vi "Main.vi"(11 "Module Admin":refnum<class "Delacor_lib_QMH_Module Admin.lvclass">) -> ()   [LabVIEW 2021, in "Test Configuration.lvlib"]
doc: "This template is based off of the Queued Message Handler design pattern and the Queued Message Handler project template that ships with LabVIEW.\n\nThe main difference is that the queue is private to this module and communication between modules is performed via Broadcast and Request events.\n\nRequest events are wrapped in public API methods and are handled in the Event Handling Loop (EHL) of this VI. Any module can register for Broadcast events sent by this module. The EHL generates messages based on user interface actions.\n\nThe Message Handling Loop (MHL) processes messages generated by the EHL, or by other messages. The messages are string values, so new messages can be added easily to the Message Cases case structure in the MHL. Each message cluster can also provide an optional value for Message Data, which is a variant that can be converted to whatever message-specific data is required.\n_____\nBased on DQMH Project Template 7.0.1.1316."
uses:
  Test Configuration.lvlib
  <vilib>/Delacor/Delacor QMH/Libraries/Module Admin_class/Delacor_lib_QMH_Module Admin.lvclass
  Module Data--cluster.ctl
  <vilib>/Wovalab/Utilities/Helper Loop Periodic Timing/Helper Loop Periodic Timing.lvclass/Helper Loop Periodic Timing.ctl
  Host-Control's/Module ID Action Enum.ctl
  <vilib>/Delacor/Delacor QMH/Libraries/Message Queue_class/Delacor_lib_QMH_Message Queue.lvclass/Delacor_lib_QMH_Message Queue.ctl
  Stop Argument--cluster.ctl
  <vilib>/Delacor/Delacor QMH/Libraries/Module Admin_class/Delacor_lib_QMH_Module Admin.lvclass/Delacor_lib_QMH_Module Admin.ctl
  <vilib>/Utility/miscctls.llb/LVPointTypeDef.ctl
  Host-Control's/DTT Test folder Name's.ctl
  <vilib>/Delacor/Delacor QMH/Libraries/Message Queue_class/Delacor_lib_QMH_Enqueue Message (Single).vi
  <vilib>/Delacor/Delacor QMH/Libraries/Module Admin_class/Delacor_lib_QMH_Get External Launch.vi
  <vilib>/Wovalab/Utilities/Helper Loop Periodic Timing/U32 Max Value--constant.vi
  <vilib>/Wovalab/Utilities/Helper Loop Periodic Timing/Update Last Execution Time.vi
  <vilib>/Utility/traverseref.llb/TRef Get All FP References.vi
  <vilib>/Utility/traverseref.llb/Get GObject Label.vi
  <vilib>/Wovalab/Utilities/Helper Loop Periodic Timing/Helper Loop Periodic Timing.lvclass
  <vilib>/Delacor/Delacor QMH/Libraries/Message Queue_class/Delacor_lib_QMH_Message Queue.lvclass
  Main-Module/Host Main.lvlib
  RT Acquisition Engine/RT Acquisition Engine.lvlib
  <userlib>/_OpenG.lib/appcontrol/appcontrol.llb/openg_application_control.lvlib
panel:
  in  "Proceed":bool
  in  "Open Auto-Seq Config File":bool
  out "Auto Sequence Configuration File":path
  in  "Open sb-RIO Config Folder":bool
  out "Airbag Configuration File":path
  in  "Open Crio Config Folder":bool
  out "Capsule Configuration File":path
  out "Capsule-3":bool
  out "Capsule-4":bool
  out "Capsule-2":bool
  in  "Auto ?":bool
  in  "EM valve Delay (mS)":u32=1000
  out "sb-RIO":bool
  out "Capsule-1":bool
  out "Release":bool
  out "Safety":bool
  in  "Hardware Status check":bool
  in  "Gate valve Delay (mS)":u32=1000
  in  "Data Logging Duration (Sec)":dbl=20.0 min=10.0 max=70.0
  out "error out":errorcluster
  out "Status":string
  in  "Simulate MHL Error":bool
  in  "Simulate EHL Error":bool
  # "IIT M Drop Tower Test System"
  # "TEST CONFIGURATION"
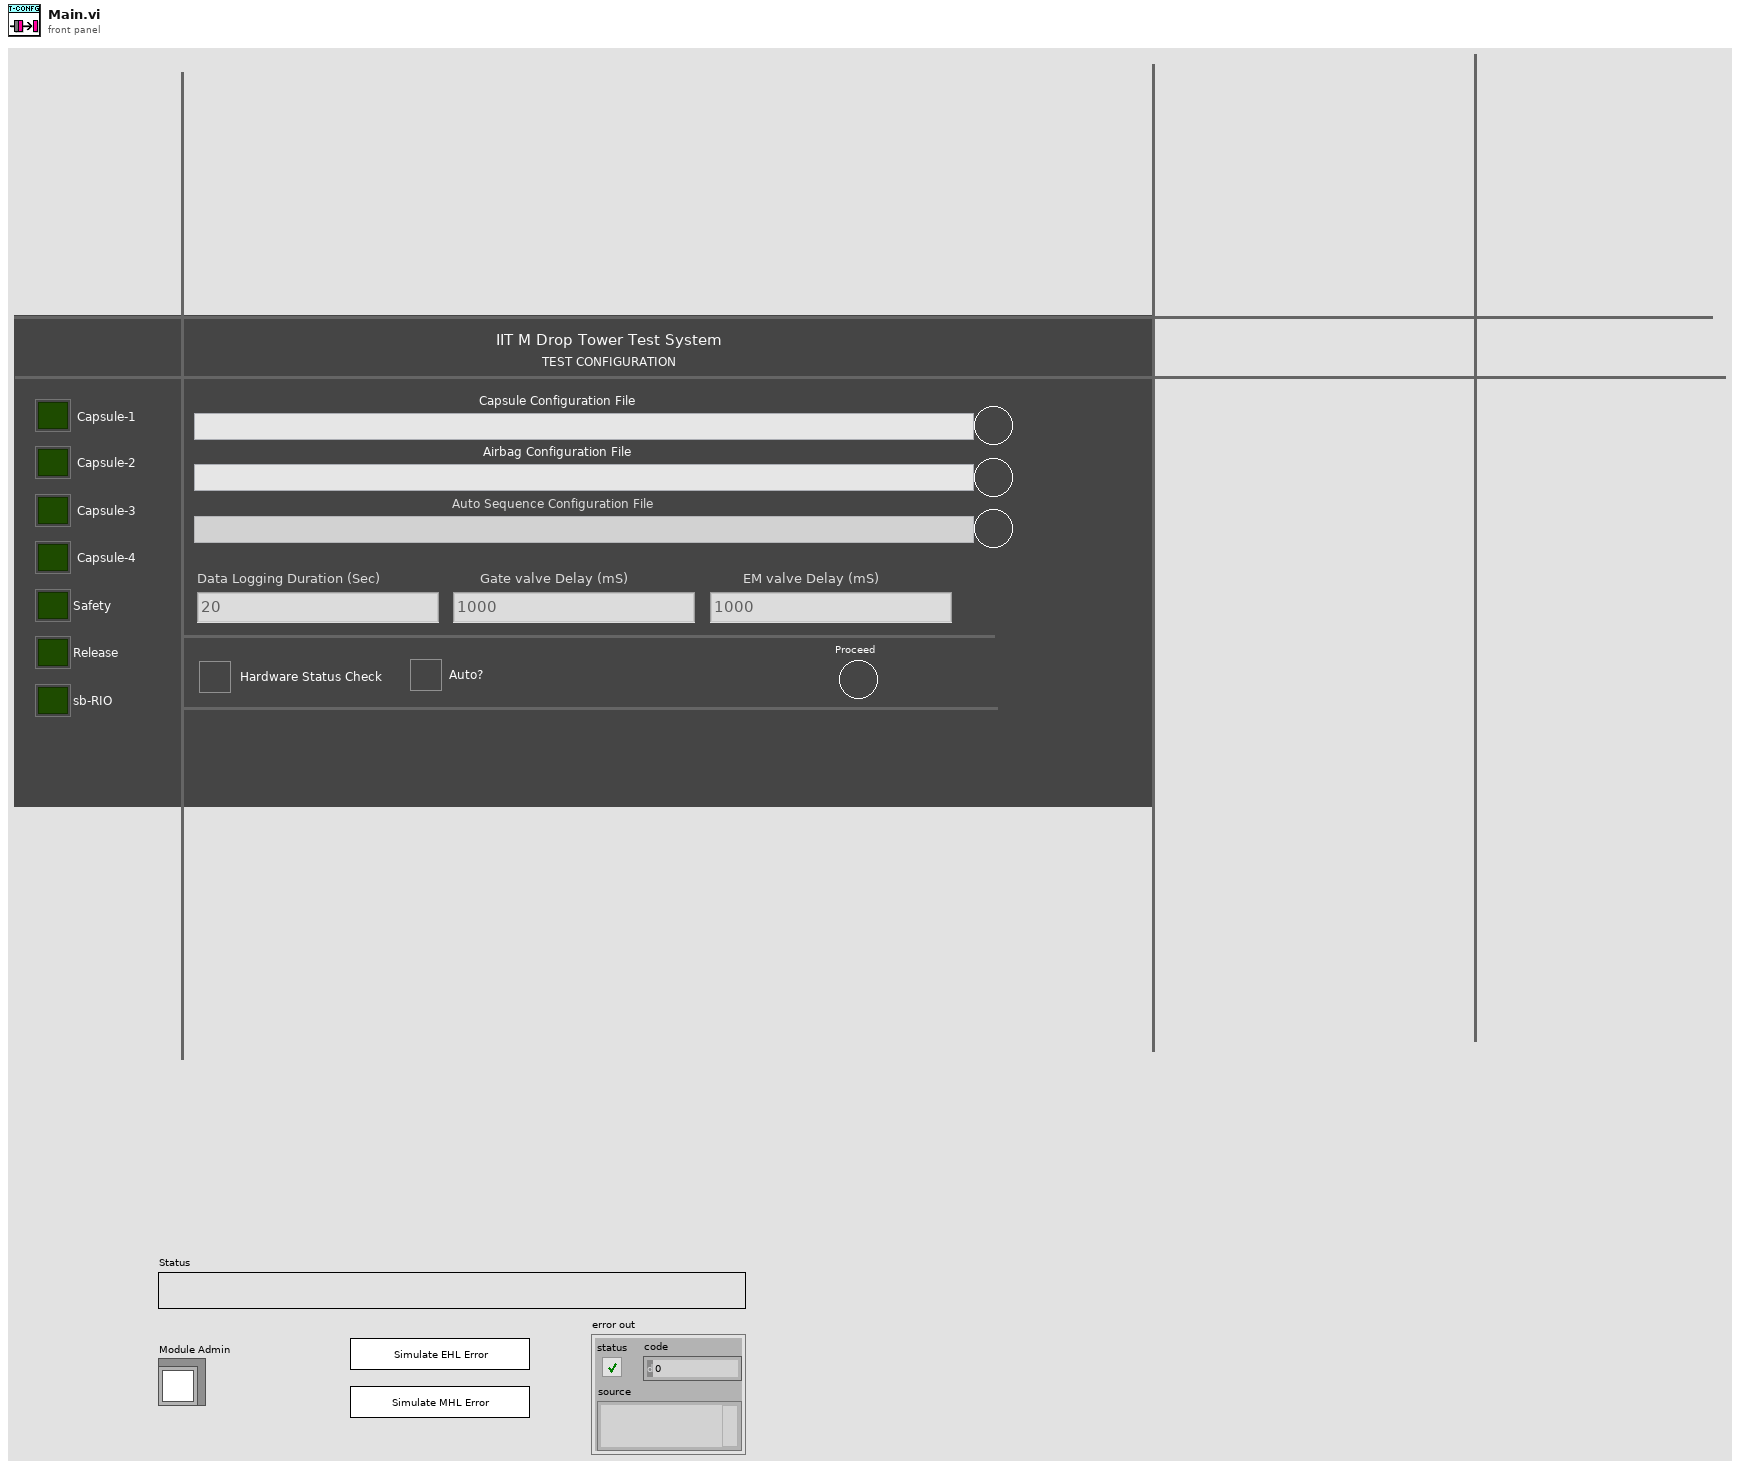
[diagram p1: front panel]
types:
  T1 = typedef "Test Configuration.lvlib/Request Events--cluster.ctl" = cluster{"Stop Module":refnum<user-event>, "Show Panel":refnum<user-event>, "Hide Panel":refnum<user-event>, "Get Module Execution Status":refnum<user-event>, "Show Diagram":refnum<user-event>}
  T2 = typedef "Test Configuration.lvlib/Module Data--cluster.ctl" = cluster{"Status":string, "Channel config Stating Path":path, "Auto-Seq config Stating Path":path, "c-RIO Tx Data":cluster{"cRIO-Module ID":i32, "AI-Config Data":string[], "AO-Config Data":string[], "DI-Config Data":string[], "DO-Config Data":string[], "AI-Start Cmd":string[], "AO-Start Cmd":string[], "DI-Start Cmd":string[], "DO-Start Cmd":string[], "AS Config Cmd":string}, "Auto Sequence Selected?":bool, "This VI":refnum<vi>, "GUI Data's":cluster{"All Object Ref":refnum<vi>[], "All Object Label":string[]}}
  T3 = typedef "Module ID Action Enum.ctl" = enum16{"Init", "Insert", "Get a ID", "Get all ID"}
  T4 = enum32{"invalid lock state", "Not Locked", "Locked (No Password)", "Password-protected"}
  T5 = typedef "Test Configuration.lvlib/Stop Argument--cluster.ctl" = cluster{"Origin":string, "Exit via Stop Module Req?":bool, "Wait for Module to stop?":bool}
  T6 = typedef "LVPointTypeDef.ctl" = cluster{"Horizontal":i16, "Vertical":i16}
  T7 = enum32{"Invalid", "Standard", "Closed", "Hidden", "Minimized", "Maximized"}
  T8 = typedef "DTT Test folder Name's.ctl" = enum16{"Event Log", "Auto Sequence Configuration", "Channel Configuration's", "Test Data's"}
  T9 = enum8{"Enabled", "Disabled", "Disabled and Grayed Out"}
  T10 = typedef "RT Acquisition Engine.lvlib/Broadcast Events--cluster.ctl" = cluster{"Module Did Init":refnum<user-event>, "Status Updated":refnum<user-event>, "Error Reported":refnum<user-event>, "Module Did Stop":refnum<user-event>, "Update Module Execution Status":refnum<user-event>, "RT Connection Status":refnum<user-event>, "Tx RT Hardware Info":refnum<user-event>, "DO Data's":refnum<user-event>, "AI-Info":refnum<user-event>, "Logging Completed":refnum<user-event>}
  T11 = typedef "HW Name Enum.ctl" = enum16{"Capsule-1", "Capsule-2", "Capsule-3", "Capsule-4", "sb-RIO", "Safety", "Release"}
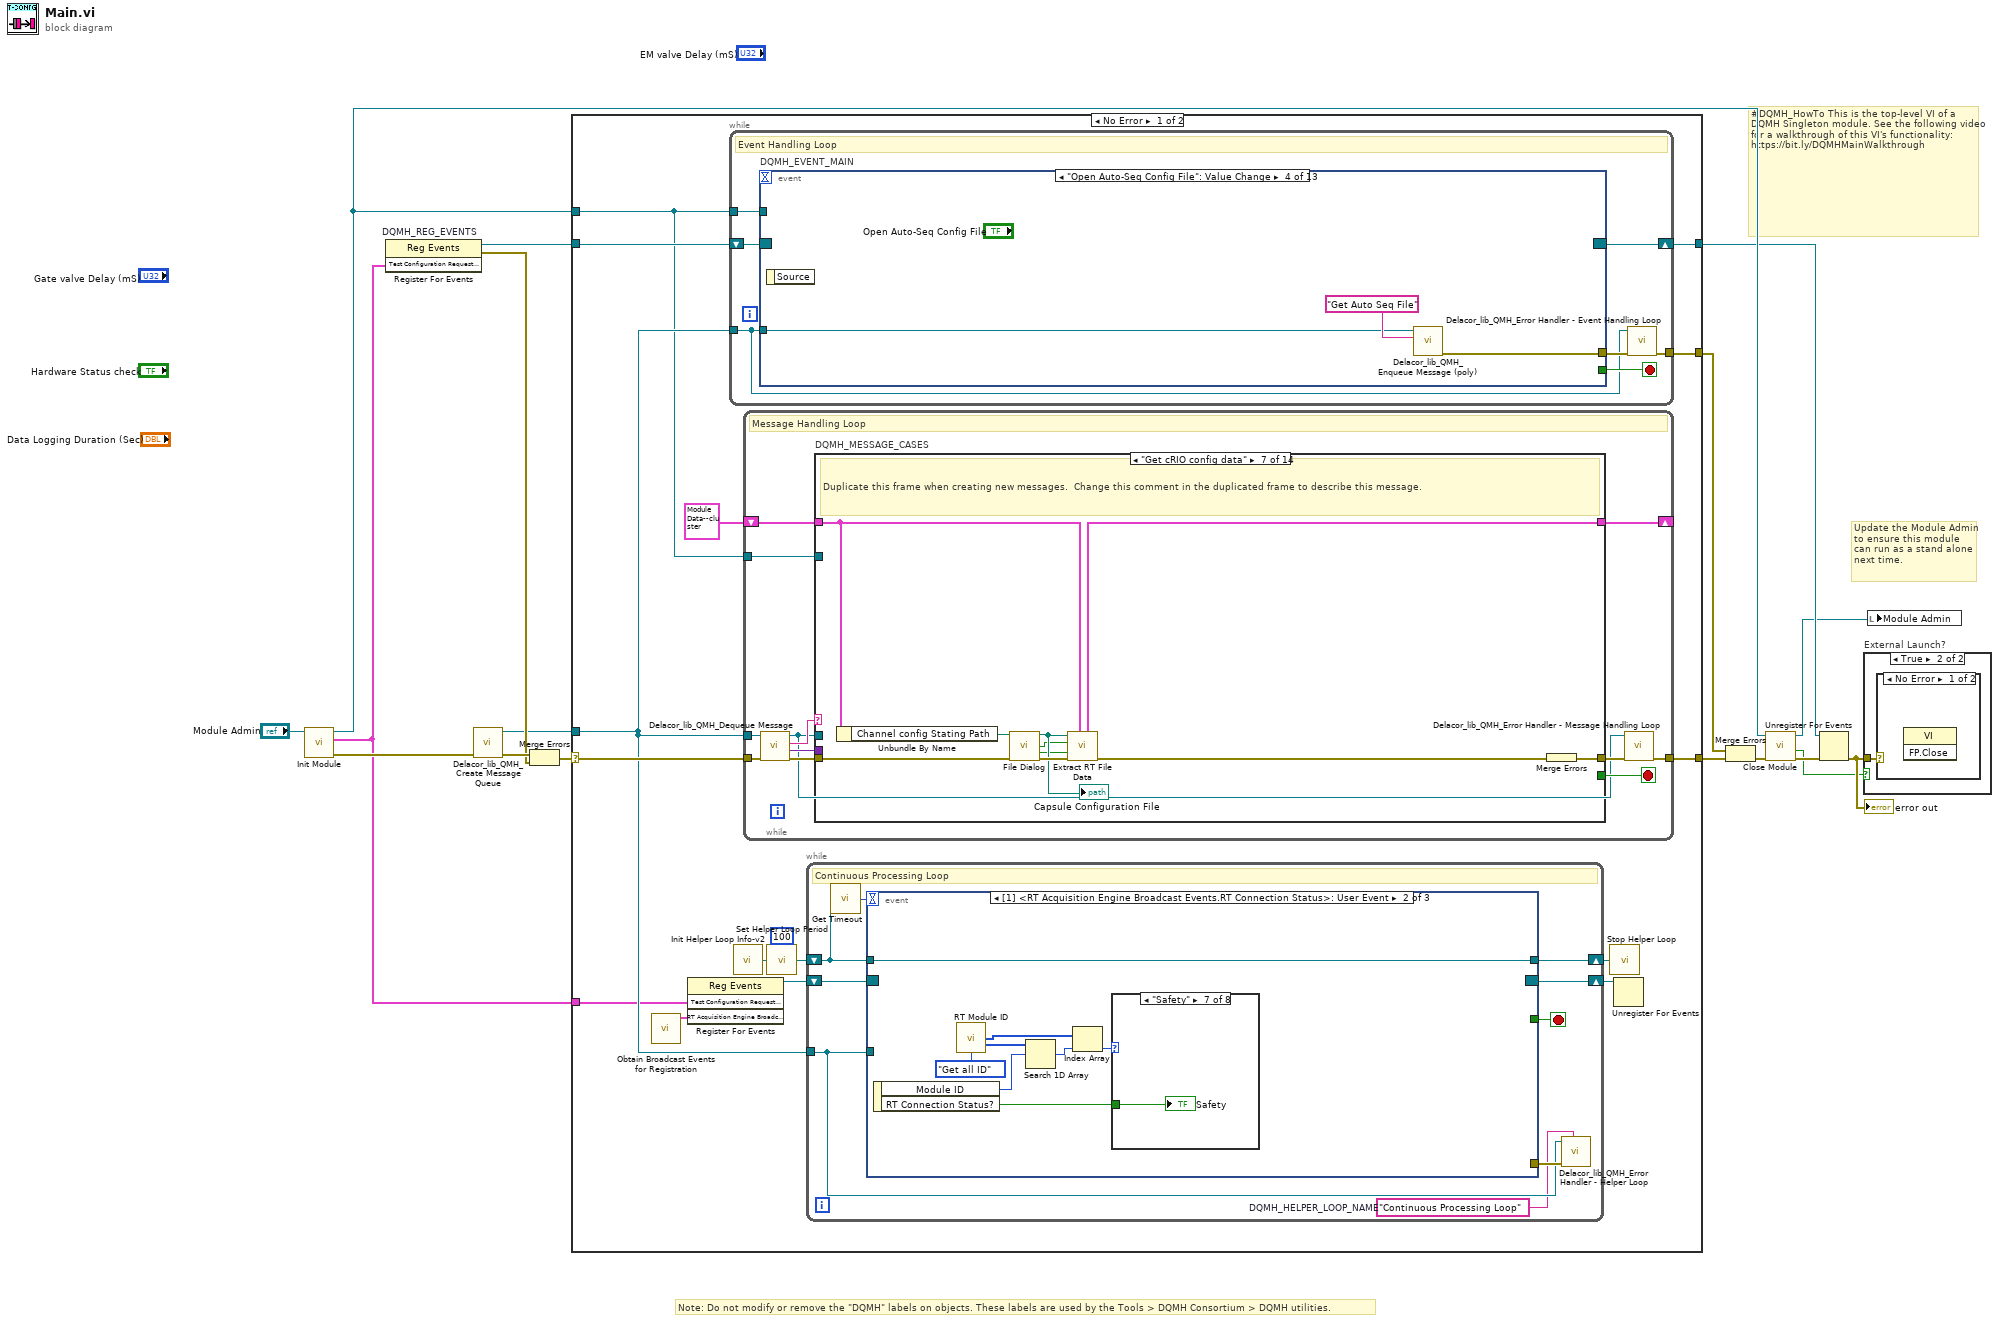
[diagram p0: block diagram]
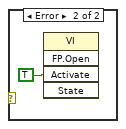
[diagram p3: hidden frame]
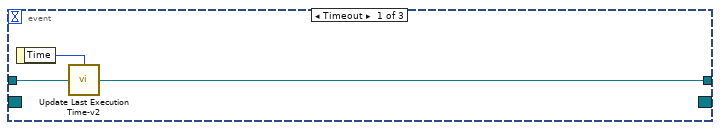
[diagram p4: hidden frame]
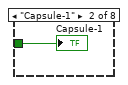
[diagram p6: hidden frame]
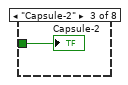
[diagram p7: hidden frame]
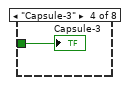
[diagram p8: hidden frame]
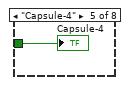
[diagram p9: hidden frame]
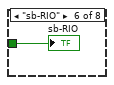
[diagram p10: hidden frame]
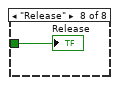
[diagram p11: hidden frame]
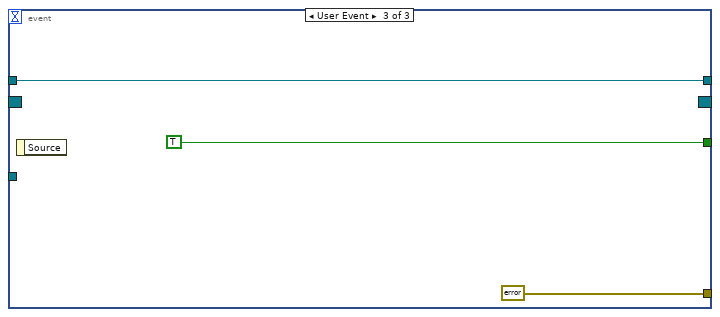
[diagram p12: hidden frame]
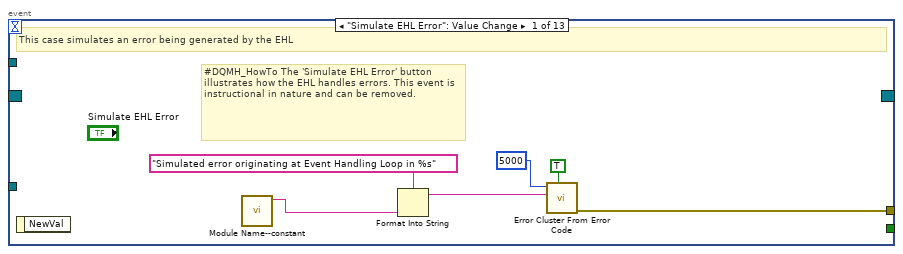
[diagram p13: hidden frame]
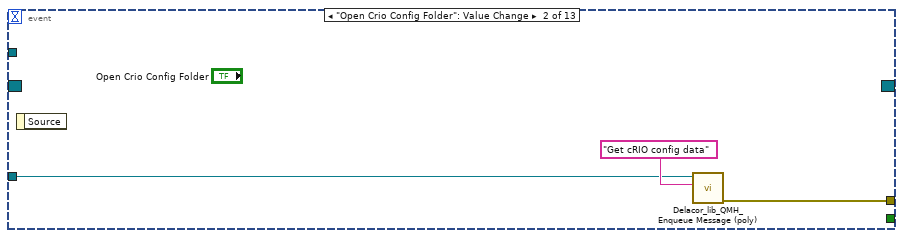
[diagram p14: hidden frame]
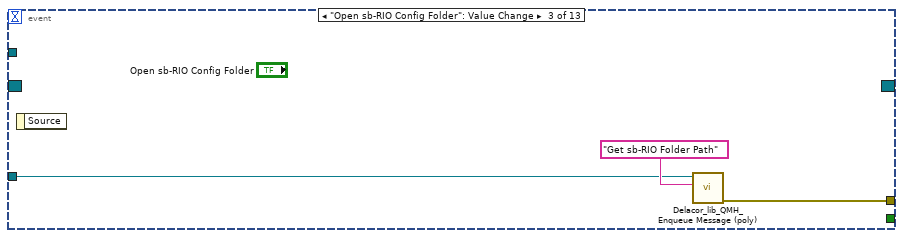
[diagram p15: hidden frame]
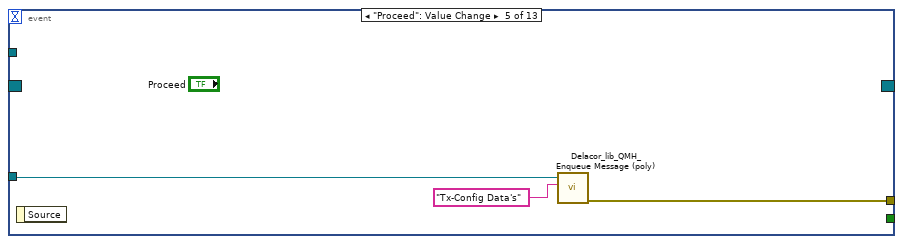
[diagram p16: hidden frame]
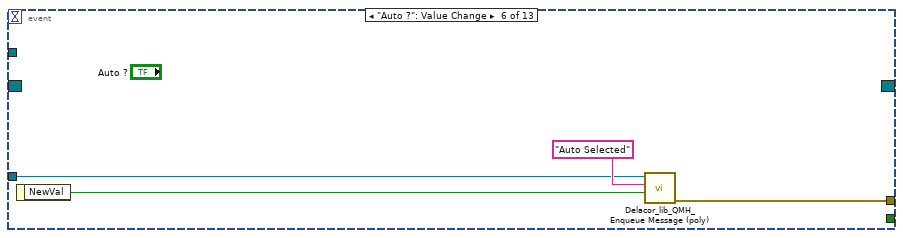
[diagram p17: hidden frame]
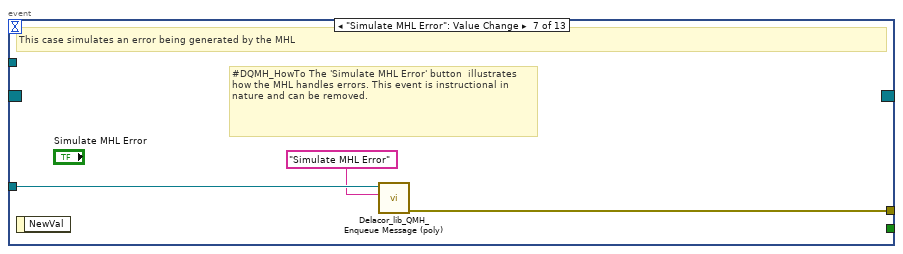
[diagram p18: hidden frame]
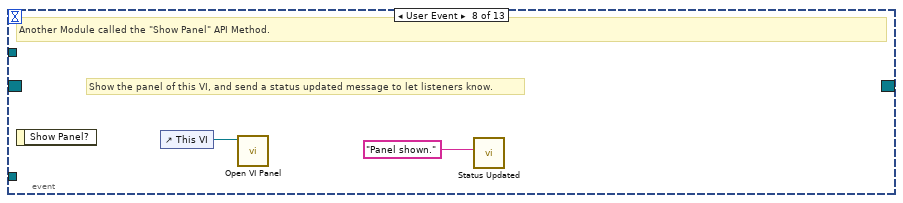
[diagram p19: hidden frame]
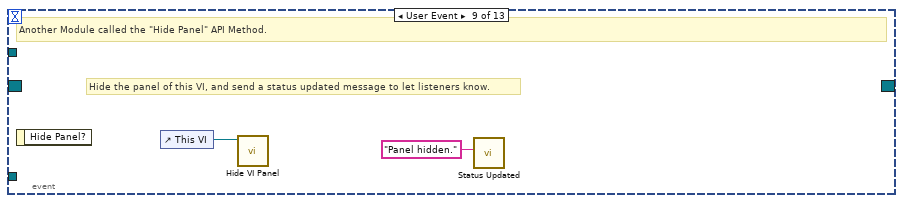
[diagram p20: hidden frame]
diagram:
  # "#DQMH_HowTo This is the top-level VI of a DQMH Singleton module. See the following video for a walkthrough of this VI's functionality: https://bit.ly/DQMHMainWalkthrough"
  # "Note: Do not modify or remove the \"DQMH\" labels on objects. These labels are used by the Tools > DQMH Consortium > DQMH utilities."
  # "Update the Module Admin to ensure this module can run as a stand alone next time."
  n1 = call "Init Module.vi"("Singleton Module Admin in"="Module Admin") -> ("error out"=w16:errorcluster, "Test Configuration Request Events"=w1:T1, "Singleton Module Admin out"=w8:refnum<class "Delacor_lib_QMH_Module Admin.lvclass">)  [unwired: 8 in]
  n2 = register-events "DQMH_REG_EVENTS"(w1) -> (reference out=w6:refnum<event-registration>, error out=w9:errorcluster)  [unwired: 2 in]
  n3 = call <vilib>:"Delacor_lib_QMH_Create Message Queue.vi"("error in"=w16) -> ("error out"=w11:errorcluster, "Message Queue"=w5:refnum<class "Delacor_lib_QMH_Message Queue.lvclass">)  [unwired: 9 in]
  n4 = Merge Errors(w11, w9) -> (w10:errorcluster)
  n5 = case shown="No Error" w10 {
    selector: w10 -> [w31 w340]
    tunnel: [w33 w339] -> w17
    tunnel: [w30 w338] -> w7
    tunnel: w6 -> [w28 w338]
    tunnel: w5 -> [w27 w333]
    tunnel: [w32 _] -> w14
    tunnel: w8 -> [w26 w334]
    tunnel: w1 -> [w25 _]
    frame No Error {
      n6 = call "Obtain Broadcast Events for Registration.vi"() -> ("RT Acquisition Engine Broadcast Events"=w22:T10)  [unwired: 9 in, 2 out]
      n7 = register-events ("DQMH_HELPER_REGFOREVENTS")(w25, w22) -> (reference out=w23:refnum<event-registration>)  [unwired: 2 in, 1 out]
      n8 = while {
        tunnel: w27 -> [w64]
        shift-right: [w67] -> w30
        shift-left: w28 -> [w68]
        tunnel: [w69] -> w32
        tunnel: w26 -> [w65]
        stop <- w66 stop-if-true
        # "Event Handling Loop"
        n9 = event "DQMH_EVENT_MAIN" shown="[3] \"Open Auto-Seq Config File\": Value Change" {
          selector: w68 -> [_ _ _ _ _ _ _ _ _ _ _ _ _]
          dyn-events: [_ _ _ _ _ _ _ _ _ _ _ _ _] -> w67
          timeout: _ -> [_ _ _ _ _ _ _ _ _ _ _ _ _]
          tunnel: [_ _ _ _ _ _ _ _ _ _ _ TRUE ("Discard?") _] -> w66
          tunnel: w64 -> [_ w78 w80 w83 w86 w90 w94 _ _ _ _ w113 w127]
          tunnel: [w76 w77 w81 w84 w87 w91 w95 _ _ w101 _ w123 w129] -> w70
          tunnel: w65 -> [_ _ _ _ _ _ _ _ _ _ _ _ w126]
          event "Simulate EHL Error": Value Change {
            # "#DQMH_HowTo The 'Simulate EHL Error' button  illustrates how the EHL handles errors. This event is instructional in nature and can be removed."
            # "This case simulates an error being generated by the EHL"
            n10 = event-data() -> ()  [unwired: 1 in, 1 out]
            n11 = call "Module Name--constant.vi"() -> ("Module Name"=w73:string)  [unwired: 11 in]
            n12 = Format Into String(format string="Simulated error originating at Event Handling Loop in %s", w73) -> (resulting string=w74:string)  [unwired: 2 in, 1 out]
            n13 = call <vilib>:"Error Cluster From Error Code.vi"("show call chain? (False)"=TRUE, "error message (\"\")"=w74, "error code (0)"=5000) -> ("error out"=w76:errorcluster)  [unwired: 6 in]
          }
          event "Open Crio Config Folder": Value Change {
            n14 = event-data() -> ()  [unwired: 1 in, 1 out]
            n15 = call-poly <vilib>:"Delacor_lib_QMH_Enqueue Message (poly).vi"("Message"="Get cRIO config data", "Message Queue in"=w78) -> ("error out"=w77:errorcluster)  [unwired: 8 in, 1 out]
          }
          event "Open sb-RIO Config Folder": Value Change {
            n16 = event-data() -> ()  [unwired: 1 in, 1 out]
            n17 = call-poly <vilib>:"Delacor_lib_QMH_Enqueue Message (poly).vi"("Message"="Get sb-RIO Folder Path", "Message Queue in"=w80) -> ("error out"=w81:errorcluster)  [unwired: 8 in, 1 out]
          }
          event "Open Auto-Seq Config File": Value Change {
            n18 = event-data() -> ()  [unwired: 1 in, 1 out]
            n19 = call-poly <vilib>:"Delacor_lib_QMH_Enqueue Message (poly).vi"("Message"="Get Auto Seq File", "Message Queue in"=w83) -> ("error out"=w84:errorcluster)  [unwired: 8 in, 1 out]
          }
          event "Proceed": Value Change {
            n20 = event-data() -> ()  [unwired: 1 in, 1 out]
            n21 = call-poly <vilib>:"Delacor_lib_QMH_Enqueue Message (poly).vi"("Message"="Tx-Config Data's", "Message Queue in"=w86) -> ("error out"=w87:errorcluster)  [unwired: 8 in, 1 out]
          }
          event "Auto ?": Value Change {
            n22 = event-data() -> ("NewVal"=w89:bool)  [unwired: 1 in]
            n23 = call-poly <vilib>:"Delacor_lib_QMH_Enqueue Message (poly).vi"("Message Data"=w89, "Message"="Auto Selected", "Message Queue in"=w90) -> ("error out"=w91:errorcluster)  [unwired: 7 in, 1 out]
          }
          event "Simulate MHL Error": Value Change {
            # "#DQMH_HowTo The 'Simulate MHL Error' button  illustrates how the MHL handles errors. This event is instructional in nature and can be removed."
            # "This case simulates an error being generated by the MHL"
            n24 = event-data() -> ()  [unwired: 1 in, 1 out]
            n25 = call-poly <vilib>:"Delacor_lib_QMH_Enqueue Message (poly).vi"("Message"="Simulate MHL Error", "Message Queue in"=w94) -> ("error out"=w95:errorcluster)  [unwired: 8 in, 1 out]
          }
          event User Event {
            # "Show the panel of this VI, and send a status updated message to let listeners know."
            # "Another Module called the \"Show Panel\" API Method."
            n26 = event-data() -> ()  [unwired: 1 in, 1 out]
            n27 = control-ref of="This VI"() -> (w97:refnum<vi>)
            n28 = call "Open VI Panel.vi"("VI"=w97) -> ()  [unwired: 10 in, 1 out]
            n29 = call "Status Updated.vi"("Status"="Panel shown." ("format string")) -> ()  [unwired: 10 in, 1 out]
          }
          event User Event {
            # "Hide the panel of this VI, and send a status updated message to let listeners know."
            # "Another Module called the \"Hide Panel\" API Method."
            n30 = event-data() -> ()  [unwired: 1 in, 1 out]
            n31 = control-ref of="This VI"() -> (w99:refnum<vi>)
            n32 = call "Hide VI Panel.vi"("VI"=w99) -> ()  [unwired: 10 in, 1 out]
            n33 = call "Status Updated.vi"("Status"="Panel hidden." ("format string")) -> ()  [unwired: 10 in, 1 out]
          }
          event User Event {
            # "Another Module called the \"Get Module Execution Status\" API Method."
            n34 = event-data() -> ()  [unwired: 1 in, 1 out]
            n35 = call "Update Module Execution Status.vi"("Running?"=TRUE) -> ("error out"=w101:errorcluster)  [unwired: 10 in]
          }
          event User Event {
            # "Another Module called the \"Show Diagram\" API Method. This event is used for debugging."
            n36 = event-data() -> ()  [unwired: 1 in, 1 out]
            n37 = disable-structure shown="RUN_TIME_ENGINE==False" {
              frame condition #0 (active) {
                # "functionality not available in exe"
                n38 = invoke on="Invoke Node" class="VI" method="Lock State.Get"() -> (error out=w107:errorcluster, "Get Lock State"=w106:T4, "pwd in cache"=w103:bool)  [unwired: 4 in, 1 out]
                n39 = Equal?(x=T4."Password-protected", y=w106) -> (x = y?=w104:bool)
                n40 = Compound Arithmetic op=AND(w104, invert w103) -> (w102:bool)
                n41 = case shown="False" w102 {
                  tunnel: w107 -> [w110 _]
                  frame False {
                    n42 = property on="Property Node" class="VI"(error in=w110, "BDWin.Open"=TRUE ("Block Diagram Window:Open")) -> ()  [unwired: 1 in, 2 out]
                    n43 = call "Status Updated.vi"("Status"="Block Diagram shown." ("format string")) -> ()  [unwired: 10 in, 1 out]
                  }
                  frame True {
                    # "Password-protected VI, and the password is not in the cache. Do not show the diagram."
                  }
                }
              }
              frame condition #1 {
              }
            }
          }
          event User Event {
            # "The Stop Module Event can get fired from the Exit message in the MHL. The queue gets destroyed in that case. If the queue no longer exists, the Enqueue Exit as a priority message will return error 1. It is safe to ignore, because the module is already exiting."
            # "Another Module called the \"Stop Module\" API Method  or the Message Handling Loop below."
            n44 = event-data() -> ("Origin"=w120:string, "Exit via Stop Module Req?"=w116:bool, "Wait for Module to stop?"=w115:bool)  [unwired: 1 in]
            n45 = local write "Status"(w120) -> ()
            n46 = Bundle By Name(cluster=T5 {"Origin"="", "Exit via Stop Module Req?"=FALSE, "Wait for Module to stop?"=FALSE} ("Stop Argument"), "Exit via Stop Module Req?"=w116, "Wait for Module to stop?"=w115) -> (w114:T5)
            n47 = call-dynamic "Delacor_lib_QMH_Flush Messages.vi"("Message Queue in"=w113) -> ("error out"=w111:errorcluster, "Message Queue out"=w112:refnum<class "Delacor_lib_QMH_Message Queue.lvclass">)  [unwired: 7 in, 2 out]
            n48 = call-poly <vilib>:"Delacor_lib_QMH_Enqueue Message (poly).vi"("Priority Message? (F)"=TRUE, "error in"=w111, "Message Data"=w114, "Message"="Exit", "Message Queue in"=w112) -> ("error out"=w124:errorcluster)  [unwired: 5 in, 1 out]
            n49 = call <vilib>:"Clear Errors.vi"("error in (no error)"=w124, "specific error code to clear (0: all)"=1) -> ("error out"=w123:errorcluster)  [unwired: 4 in, 1 out]
          }
          event Panel Close? {
            w128 = TRUE  # Discard the event, the MHL is responsible for closing and stopping this VI.
            # "Hide the panel or send the 'Exit' message if the user clicks the 'X' on the module main VI panel."
            n50 = event-data() -> ()  [unwired: 1 in, 1 out]
            n51 = property on="Property Node" class="Module Admin"(reference=w126) -> ("Accessors:External Launch"=w125:bool)  [unwired: 1 in, 2 out]
            n52 = case shown="True" w125 {
              tunnel: w127 -> [_ w136]
              tunnel: [_ w137] -> w129
              frame True {
                # "If externally launched, clicking the 'X' hides the panel, but doesn't close it."
                n53 = control-ref of="This VI"() -> (w133:refnum<vi>)
                n54 = call "Hide VI Panel.vi"("VI"=w133) -> ("error out"=w131:errorcluster)  [unwired: 10 in]
                n55 = call "Status Updated.vi"("error in"=w131, "Status"="Panel hidden." ("format string")) -> ()  [unwired: 9 in, 1 out]
                n56 = call "Hide Panel.vi"() -> ("error out"=w130:errorcluster)  [unwired: 11 in]
                n57 = call "Show Panel.vi"("error in"=w130) -> ()  [unwired: 10 in, 1 out]
              }
              frame False {
                # "If run as a stand-alone VI, clicking the panel 'X' stops the VI."
                n58 = call-poly <vilib>:"Delacor_lib_QMH_Enqueue Message (poly).vi"("Priority Message? (F)"=TRUE, "Message"="Exit", "Message Queue in"=w136) -> ("error out"=w137:errorcluster)  [unwired: 7 in, 1 out]
              }
            }
            n59 = event-data ("Event Filter Node")("Discard?"=w128) -> ()  [unwired: 1 in, 1 out]
          }
        }
        n60 = call-dynamic "Delacor_lib_QMH_Error Handler - Event Handling Loop.vi"("error in"=w70, "Message Queue in"=w64) -> ("dup error in"=w69:errorcluster)  [unwired: 8 in, 1 out]
      }
      n61 = call <vilib>:"Init Helper Loop Info-v2.vi"() -> ("Helper Loop Periodic Timing"=w20:refnum<class "Helper Loop Periodic Timing.lvclass">)  [unwired: 1 in]
      n62 = while {
        tunnel: w27 -> [w138]
        shift-right: [w146] -> _
        shift-left: T2 {"Status"="", "Channel config Stating Path"=path "", "Auto-Seq config Stating Path"=path "", "c-RIO Tx Data"={"cRIO-Module ID"=0, "AI-Config Data"=[], "AO-Config Data"=[], "DI-Config Data"=[], "DO-Config Data"=[], "AI-Start Cmd"=[], "AO-Start Cmd"=[], "DI-Start Cmd"=[], "DO-Start Cmd"=[], "AS Config Cmd"=""}, "Auto Sequence Selected?"=FALSE, "This VI"=refnum, "GUI Data's"={"All Object Ref"=[], "All Object Label"=[]}} ("Data Cluster") -> [w147]
        tunnel: w31 -> [w149]
        tunnel: [w141] -> w33
        tunnel: w26 -> [w142]
        stop <- w145 stop-if-true
        # "Message Handling Loop"
        n63 = call-dynamic "Delacor_lib_QMH_Dequeue Message.vi"("error in"=w149, "Message Queue in"=w138) -> ("error out"=w148:errorcluster, "Message Data"=w143:variant, "Message"=w144:string, "Message Queue out"=w139:refnum<class "Delacor_lib_QMH_Message Queue.lvclass">)  [unwired: 6 in]
        n64 = case "DQMH_MESSAGE_CASES" shown="\"Get cRIO config data\"" w144 {
          selector: w144 -> [_ _ _ _ _ _ _ _ _ _ _ _ _ w328]
          tunnel: w139 -> [w156 _ _ _ _ _ _ _ _ _ _ w294 w316 _]
          tunnel: w148 -> [w178 w182 w225 w228 w238 w244 w258 w267 w277 w281 w290 w301 w322 w331]
          tunnel: [w157 w186 w225 w227 w239 w245 w259 w269 w279 w281 w289 w297 w317 w332] -> w140
          tunnel: w147 -> [w168 w185 w224 w226 w235 w241 w251 w261 w276 w280 w287 w296 w315 w329]
          tunnel: [w167 w181 w224 w226 w234 w240 w250 w260 w275 w280 w287 w296 w315 w329] -> w146
          tunnel: [_ _ _ _ _ _ _ _ _ _ _ _ w314 _] -> w145
          tunnel: w143 -> [_ _ _ _ w237 _ _ _ _ _ _ w295 w313 _]
          tunnel: w142 -> [w169 _ _ _ _ _ _ _ _ _ _ w293 w308 _]
          frame "Initialize" {
            w163 = "Initial Message" ("Initial Message")
            # "Initialize - Any operation that needs to be done before the module can receive messages. Synchronize Caller Events.vi will inform Start Module.vi that the module has launched and is ready to receive messages. Module Did Init.vi will broadcast that the module initialized."
            n65 = call "Synchronize Caller Events.vi"("error in"=w178, "Singleton Module Admin in"=w169) -> ("error out"=w177:errorcluster, "Singleton Module Admin out"=w164:refnum<class "Delacor_lib_QMH_Module Admin.lvclass">)  [unwired: 8 in]
            n66 = property on="Property Node" class="Module Admin"(reference=w164) -> ("Accessors:External Launch"=w173:bool)  [unwired: 1 in, 2 out]
            n67 = Select(t=T7."Hidden" ("State"), s=w173, f=T7."Standard" ("State")) -> (s? t:f=w170:T7)
            n68 = control-ref of="This VI"() -> (w150:refnum<vi>)
            n69 = call "Module Name--constant.vi"() -> ("Module Name"=w176:string)  [unwired: 11 in]
            n70 = property on="Property Node" class="VI"(reference=w150, "Front Panel.Title"=w176) -> (reference out=w175:refnum<vi>, error out=w180:errorcluster)  [unwired: 1 in]
            n71 = call "Module Name--constant.vi"() -> ("Module Name"=w165:string)  [unwired: 11 in]
            n72 = invoke on="Invoke Node" class="VI" method="FP.Open"(reference=w175, error in=w180, "State"=w170) -> (reference out=w174:refnum<vi>, error out=w179:errorcluster)  [unwired: 2 in, 3 out]
            n73 = call "Module Did Init.vi"("error in"=w177, "Initialized?"=TRUE, "Origin"=w165) -> ("error out"=w159:errorcluster)  [unwired: 8 in]
            n74 = Bundle By Name(cluster=w168, "Status"=w163, "This VI"=w150) -> (w167:T2)
            n75 = invoke on="Invoke Node" class="VI" method="FP.Center"(reference=w174, error in=w179) -> (reference out=w155:refnum<vi>, error out=w154:errorcluster)  [unwired: 1 in, 1 out]
            n76 = property on="Pane" class="Pane"("Origin"=T6 {"Horizontal"=0, "Vertical"=0}) -> ()  [unwired: 2 in, 2 out]
            n77 = invoke class="VI" method="Default Vals.Reinit All"(reference=w155, error in=w154) -> (reference out=w152:refnum<vi>, error out=w151:errorcluster)  [unwired: 1 in, 1 out]
            n78 = call-poly <vilib>:"Delacor_lib_QMH_Enqueue Message (poly).vi"("error in"=w159, "Message"="Init-1", "Message Queue in"=w156) -> ("error out"=w158:errorcluster)  [unwired: 7 in, 1 out]
            n79 = call <vilib>:"Clear Errors.vi"("error in (no error)"=w151) -> ("error out"=w153:errorcluster)  [unwired: 5 in, 1 out]
            n80 = call <userlib>:"Fit VI window to Largest Dec__ogtk.vi"("error in (no error)"=w153, "VI Ref (calling VI)"=w152) -> ("error out"=w161:errorcluster)  [unwired: 4 in, 1 out]
            n81 = call <vilib>:"Clear Errors.vi"("error in (no error)"=w161) -> ()  [unwired: 5 in, 2 out]
            n82 = Merge Errors(w158) -> (w157:errorcluster)
            "Status" <- w163
          }
          frame "Init-1" {
            # "Duplicate this frame when creating new messages.  Change this comment in the duplicated frame to describe this message."
            n83 = for {
              N: 11 -> [_]
              shift-right: [w191] -> w181
              shift-left: w185 -> [w190]
              shift-right: [w189] -> w183
              shift-left: w182 -> [w188]
              i -> [w187]
              n84 = case shown="0, Default" w187 {
                tunnel: [w192 w199 w203 w208 w210 w212 w214 w216 w218 w220 w223] -> w191
                tunnel: w190 -> [w195 w199 w204 w208 w210 w212 w214 w216 w218 w220 w223]
                tunnel: [w197 w198 w206 w207 w209 w211 w213 w215 w217 w219 w222] -> w189
                tunnel: w188 -> [w197 w198 w206 w207 w209 w211 w213 w215 w217 w219 w222]
                frame 0, Default {
                  n85 = Unbundle By Name(w195) -> ("This VI"=w196:refnum<vi>)
                  n86 = call "GUI-Get all FP Ctrl & Indi Label and Ref.vi"("Respected VI Ref"=w196) -> ("All Object Label"=w193:string[], "All Object Ref"=w194:refnum<vi>[])  [unwired: 9 in]
                  n87 = Bundle By Name(cluster=w195, "GUI Data's.All Object Ref"=w194, "GUI Data's.All Object Label"=w193) -> (w192:T2)
                }
                frame 1 {
                }
                frame 2 {
                  n88 = call "Folder Creation.vi"("Folder Name"=DTT_Test_folder_Name's."Channel Configuration's") -> ("Selected Folder Path Out"=w202:path)  [unwired: 12 in, 2 out]
                  n89 = call "Folder Creation.vi"("Folder Name"=DTT_Test_folder_Name's."Auto Sequence Configuration") -> ("Selected Folder Path Out"=w200:path)  [unwired: 12 in, 2 out]
                  n90 = Bundle By Name(cluster=w204, "Channel config Stating Path"=w202, "Auto-Seq config Stating Path"=w200) -> (w203:T2)
                }
                frame 3 {
                }
                frame 4 {
                }
                frame 5 {
                }
                frame 6 {
                }
                frame 7 {
                }
                frame 8 {
                }
                frame 9 {
                }
                frame 10 {
                  w221 = T9."Disabled and Grayed Out" ("Disabled")
                  n91 = property on="Open Auto-Seq Config File" class="Bool"("DisabledEnum"=w221) -> ()  [unwired: 2 in, 2 out]
                  n92 = property on="Auto Sequence Configuration File" class="Path"("DisabledEnum"=w221) -> ()  [unwired: 2 in, 2 out]
                }
              }
            }
            n93 = Merge Errors(w183) -> (w186:errorcluster)
          }
          frame "---Module Specific---" {
            # "Separator -- The following cases handle messages specific to this Module."
          }
          frame "---Copy This Frame---" {
            # "Duplicate this frame when creating new messages.  Change this comment in the duplicated frame to describe this message."
            n94 = Merge Errors(w228) -> (w227:errorcluster)
          }
          frame "Auto Selected" {
            # "Duplicate this frame when creating new messages.  Change this comment in the duplicated frame to describe this message."
            n95 = Variant To Data(error in=w238, type=FALSE, Variant=w237) -> (data=w232:bool, error out=w233:errorcluster)
            n96 = Bundle By Name(cluster=w235, "Auto Sequence Selected?"=w232) -> (w234:T2)
            n97 = Select(t=T9."Enabled" ("Disabled"), s=w232, f=T9."Disabled and Grayed Out" ("Disabled")) -> (s? t:f=w229:T9)
            n98 = property on="Open Auto-Seq Config File" class="Bool"("DisabledEnum"=w229) -> ()  [unwired: 2 in, 2 out]
            n99 = property on="Auto Sequence Configuration File" class="Path"("DisabledEnum"=w229) -> ()  [unwired: 2 in, 2 out]
            n100 = Merge Errors(w233) -> (w239:errorcluster)
          }
          frame "Tx-Config Data's" {
            # "Duplicate this frame when creating new messages.  Change this comment in the duplicated frame to describe this message."
            n101 = call "Transmit Configuration Data's.vi"("Data Cluster In"=w241, "error in (no error)"=w244) -> ("error out"=w243:errorcluster, "Data Cluster Out"=w240:T2)  [unwired: 8 in]
            n102 = case shown="No Error" w243 {
              selector: w243 -> [w248 w249]
              tunnel: [w246 w249] -> w242
              frame No Error {
                n103 = call "Hide Panel.vi"("error in"=w248) -> ("error out"=w247:errorcluster)  [unwired: 10 in]
                n104 = call "Launch TP.vi"("error in"=w247) -> ("error out"=w246:errorcluster)  [unwired: 10 in]
              }
              frame Error {
              }
            }
            n105 = Merge Errors(w242) -> (w245:errorcluster)
          }
          frame "Get cRIO config data" {
            # "Duplicate this frame when creating new messages.  Change this comment in the duplicated frame to describe this message."
            n106 = Unbundle By Name(w251) -> ("Channel config Stating Path"=w257:path)
            n107 = call "File Dialog"("start path"=w257, "error in"=w258) -> ("selected path"=w255:path, "exists"=w254:bool, "cancelled"=w253:bool, "error out"=w256:errorcluster)  [unwired: 10 in]
            "Capsule Configuration File" <- w255
            n108 = call "Extract RT File Data.vi"("Data Cluster In"=w251, "Error In"=w256, "Cancellled?"=w253, "Exists?"=w254, "Folder Path"=w255) -> ("Error Out"=w252:errorcluster, "Data Cluster Out"=w250:T2)  [unwired: 5 in]
            n109 = Merge Errors(w252) -> (w259:errorcluster)
          }
          frame "Get sb-RIO Folder Path" {
            # "Duplicate this frame when creating new messages.  Change this comment in the duplicated frame to describe this message."
            n110 = Unbundle By Name(w261) -> ("Channel config Stating Path"=w268:path)
            n111 = call "File Dialog2"("start path"=w268, "error in"=w267) -> ("selected path"=w262:path, "exists"=w264:bool, "cancelled"=w263:bool, "error out"=w266:errorcluster)  [unwired: 10 in]
            "Airbag Configuration File" <- w262
            n112 = call "Extract RT File Data.vi"("Data Cluster In"=w261, "Error In"=w266, "Cancellled?"=w263, "Exists?"=w264, "Folder Path"=w262) -> ("Error Out"=w265:errorcluster, "Data Cluster Out"=w260:T2)  [unwired: 5 in]
            n113 = Merge Errors(w265) -> (w269:errorcluster)
          }
          frame "Get Auto Seq File" {
            # "Duplicate this frame when creating new messages.  Change this comment in the duplicated frame to describe this message."
            n114 = Unbundle By Name(w276) -> ("Auto-Seq config Stating Path"=w278:path)
            n115 = call "File Dialog3"("start path"=w278, "error in"=w277) -> ("selected path"=w270:path, "exists"=w272:bool, "cancelled"=w271:bool, "error out"=w274:errorcluster)  [unwired: 10 in]
            "Auto Sequence Configuration File" <- w270
            n116 = call "Extract Auto Sequence Data.vi"("Data Cluster"=w276, "error in (no error)"=w274, "Cancellled?"=w271, "Exists?"=w272, "Folder Path"=w270) -> ("error out"=w273:errorcluster, "Data Cluster Out"=w275:T2)  [unwired: 5 in]
            n117 = Merge Errors(w273) -> (w279:errorcluster)
          }
          frame "---Exit and Error Handling---" {
            # "Separator - The following cases handle errors and exit messages."
          }
          frame "Simulate MHL Error" {
            # "#DQMH_HowTo The 'Simulate MHL Error' button  illustrates how the MHL handles errors. This event is instructional in nature and can be removed."
            # "Simulate an error occurring at the MHL"
            n118 = call "Module Name--constant.vi"() -> ("Module Name"=w283:string)  [unwired: 11 in]
            n119 = Format Into String(format string="Simulated error originating at Message Handling Loop in %s", w283) -> (resulting string=w284:string)  [unwired: 2 in, 1 out]
            n120 = call <vilib>:"Error Cluster From Error Code.vi"("show call chain? (False)"=TRUE, "error message (\"\")"=w284, "error code (0)"=5001) -> ("error out"=w288:errorcluster)  [unwired: 6 in]
            n121 = Merge Errors(w290, w288) -> (w289:errorcluster)
          }
          frame "Error" {
            # "#CodeRecommended - If the module is running in standalone mode (External Launch = FALSE), this code will pop up an error dialog and call the 'Exit' message if an error occurs. Add more fine-grained error management here."
            # "Error - Check the error message data and respond accordingly. This message is sent by the \"Error Handler\" VIs at the end of each loop in this application."
            n122 = Variant To Data(error in=w301, type=errorcluster {"status"=FALSE, "code"=0, "source"=""} ("error constant"), Variant=w295) -> (data=w291:errorcluster, error out=w299:errorcluster)
            n123 = property on="Property Node" class="Module Admin"(reference=w293) -> ("Accessors:External Launch"=w292:bool)  [unwired: 1 in, 2 out]
            n124 = local write "error out"(w291) -> ()
            n125 = call "Error Reported.vi"("Error"=w291) -> ()  [unwired: 10 in, 1 out]
            n126 = case shown="False" w292 {
              tunnel: [w306 _] -> w298
              tunnel: w294 -> [w304 _]
              tunnel: w291 -> [w305 _]
              frame False {
                n127 = disable-structure shown="Default" {
                  disable-tunnel: w305 -> [w307 _]
                  frame condition #0 (active) {
                    # "If the module is running standalone, then pop up an error dialog and call the \"Exit\" message."
                    n128 = call <vilib>:"Simple Error Handler.vi"("error in (no error)"=w307) -> ()  [unwired: 4 in, 5 out]
                  }
                  frame condition #1 {
                    # "To prevent the Simple Error Handler VI from being loaded (e.g. when deploying to a Real-Time target), add the Conditional Disable Symbol \"DQMH_Disable_SEH\" to your project and set it to TRUE."
                  }
                }
                n129 = call-poly <vilib>:"Delacor_lib_QMH_Enqueue Message (poly).vi"("Priority Message? (F)"=TRUE, "Message"="Exit", "Message Queue in"=w304) -> ("error out"=w306:errorcluster)  [unwired: 7 in, 1 out]
              }
              frame True {
                # "If the module was launched externally, calling the Error Reported broadcast VI is the only action performed by the \"Error\" message. The module's caller can then process the error appropriately."
              }
            }
            n130 = Merge Errors(w299, w298) -> (w297:errorcluster)
          }
          frame "Exit" {
            w312 = 91  # 91: not all Exit messages will have an argument
            w314 = TRUE  # Stop the VI
            # "Release the message queue reference"
            # "#CodeNeeded - Add any required cleanup code here."
            # "Exit - Exit the application."
            n131 = Variant To Data(error in=w322, type=T5 {"Origin"="", "Exit via Stop Module Req?"=FALSE, "Wait for Module to stop?"=FALSE} ("Stop Argument"), Variant=w313) -> (data=w310:T5, error out=w319:errorcluster)
            n132 = call <vilib>:"Clear Errors.vi"("error in (no error)"=w319, "specific error code to clear (0: all)"=w312) -> ("error out"=w321:errorcluster)  [unwired: 4 in, 1 out]
            n133 = control-ref of="This VI"() -> (w309:refnum<vi>)
            n134 = call-dynamic "Delacor_lib_QMH_Release Message Queue.vi"("error in"=w321, "Message Queue"=w316) -> ("error out"=w320:errorcluster)  [unwired: 9 in]
            n135 = call "Handle Exit.vi"("Stop Argument"=w310, "Admin in"=w308, "VI reference"=w309) -> ("error out"=w318:errorcluster)  [unwired: 7 in, 1 out]
            n136 = Merge Errors(w320, w318) -> (w317:errorcluster)
            n137 = call "Error Reported.vi"("Error"=w317) -> ()  [unwired: 10 in, 1 out]
          }
          frame Default {
            # "'Default' case only runs if there is a message that isn't defined in any of the other cases.  Output a programming error."
            n138 = call "Module Name--constant.vi"() -> ("Module Name"=w327:string)  [unwired: 11 in]
            n139 = Format Into String(format string="The invalid message string \"%s\" was received in the Message Handling Loop for module \"%s\".", w328, w327) -> (resulting string=w323:string)  [unwired: 2 in, 1 out]
            n140 = call <vilib>:"Error Cluster From Error Code.vi"("show call chain? (False)"=TRUE, "error message (\"\")"=w323, "error code (0)"=1) -> ("error out"=w330:errorcluster)  [unwired: 6 in]
            n141 = Merge Errors(w331, w330) -> (w332:errorcluster)
          }
        }
        n142 = call-dynamic "Delacor_lib_QMH_Error Handler - Message Handling Loop.vi"("error in"=w140, "Message Queue in"=w139) -> ("dup error in"=w141:errorcluster)  [unwired: 8 in, 1 out]
      }
      n143 = call <vilib>:"Set Helper Loop Period.vi"("Period (ms)"=100, "Helper Loop Periodic Timing in"=w20) -> ("Helper Loop Periodic Timing out"=w21:refnum<class "Helper Loop Periodic Timing.lvclass">)  [unwired: 13 in]
      n144 = while "DQMH_HELPER_LOOP" {
        shift-right: [w42] -> w19
        shift-left: w21 -> [w35]
        shift-right: [w40] -> w24
        shift-left: w23 -> [w41]
        tunnel: w27 -> [w37]
        stop <- w39 stop-if-true
        w36 = "Continuous Processing Loop"  # DQMH_HELPER_LOOP_NAME
        # "Continuous Processing Loop"
        n145 = call <vilib>:"Get Timeout.vi"("Helper Loop Periodic Timing"=w35) -> ("Timeout (ms)"=w34:i32)  [unwired: 12 in, 2 out]
        n146 = event "DQMH_HELPER_EVENT_STRUCTURE" shown="[1] <RT Acquisition Engine Broadcast Events.RT Connection Status>: User Event" {
          selector: w41 -> [_ _ _]
          dyn-events: [_ _ _] -> w40
          timeout: w34 -> [_ _ _]
          tunnel: w35 -> [w44 w53 w63]
          tunnel: [w43 w53 w63] -> w42
          tunnel: [_ _ TRUE] -> w39
          tunnel: [_ _ errorcluster {"status"=FALSE, "code"=0, "source"=""} ("error constant")] -> w38
          tunnel: w37 -> [_ _ _]
          event Timeout {
            n147 = event-data() -> ("Time"=w45:u32)  [unwired: 1 in]
            n148 = call <vilib>:"Update Last Execution Time-v2.vi"("Time"=w45, "Helper Loop Periodic Timing in"=w44) -> ("Helper Loop Periodic Timing out"=w43:refnum<class "Helper Loop Periodic Timing.lvclass">)  [unwired: 12 in, 1 out]
          }
          event User Event {
            n149 = event-data() -> ("Module ID"=w47:i32, "RT Connection Status?"=w46:bool)  [unwired: 1 in]
            n150 = call "RT Module ID.vi"("Action"=Module_ID_Action_Enum."Get all ID") -> ("All HW Name Out"=w49:T11[], "All HW-ID Out"=w50:i32[])  [unwired: 11 in, 2 out]
            n151 = Search 1D Array(1D array=w50, element=w47) -> (index of element=w51:i32)  [unwired: 1 in]
            n152 = Index Array(array=w49, index=w51) -> (element=w48:T11)
            n153 = case shown="\"Safety\"" w48 {
              tunnel: w46 -> [_ w54 w55 w56 w57 w58 w59 w60]
              frame Default {
              }
              frame "Capsule-1" {
                "Capsule-1" <- w54
              }
              frame "Capsule-2" {
                "Capsule-2" <- w55
              }
              frame "Capsule-3" {
                "Capsule-3" <- w56
              }
              frame "Capsule-4" {
                "Capsule-4" <- w57
              }
              frame "sb-RIO" {
                "sb-RIO" <- w58
              }
              frame "Safety" {
                "Safety" <- w59
              }
              frame "Release" {
                "Release" <- w60
              }
            }
          }
          event User Event {
            n154 = event-data() -> ()  [unwired: 1 in, 1 out]
          }
        }
        n155 = call-dynamic "Delacor_lib_QMH_Error Handler - Helper Loop.vi"("Error Debug"=w36, "error in"=w38, "Message Queue in"=w37) -> ()  [unwired: 7 in, 2 out]
      }
      n156 = call <vilib>:"Stop Helper Loop.vi"("Helper Loop Periodic Timing in"=w19) -> ()  [unwired: 1 out]
      n157 = Unregister For Events(event registration refnum=w24) -> ()  [unwired: 1 in, 1 out]
    }
    frame Error {
      # "Synchronize Caller Events.vi will inform Start Module.vi that the module has launched and will let the code calling Start Module.vi register for broadcasts and would permit the caller receive the broadcast that an error occurred at launch time."
      n158 = call-dynamic "Delacor_lib_QMH_Release Message Queue.vi"("error in"=w340, "Message Queue"=w333) -> ("error out"=w339:errorcluster)  [unwired: 9 in]
      n159 = call "Synchronize Caller Events.vi"("Singleton Module Admin in"=w334) -> ("error out"=w341:errorcluster)  [unwired: 9 in, 1 out]
      n160 = call "Module Name--constant.vi"() -> ("Module Name"=w337:string)  [unwired: 11 in]
      n161 = Format Into String(format string="An error occurred during initialization. %s is no longer running.", w337) -> (resulting string=w335:string)  [unwired: 2 in, 1 out]
      n162 = Merge Errors(w339, w341) -> (w342:errorcluster)
      n163 = call "Error Reported.vi"("Additional Information"=w335, "Error"=w342) -> ()  [unwired: 9 in, 1 out]
    }
  }
  n164 = Merge Errors(w14, w17) -> (w13:errorcluster)
  n165 = call "Close Module.vi"("error in"=w13, "Module Admin in"=w8) -> ("error out"=w15:errorcluster, "External Launch"=w2:bool, "Module Admin out"=w3:refnum<class "Delacor_lib_QMH_Module Admin.lvclass">)  [unwired: 7 in]
  n166 = Unregister For Events(event registration refnum=w7, error in=w15) -> (error out=w12:errorcluster)
  "error out" <- w12
  n167 = case "External Launch?" shown="True" w2 {
    tunnel: w12 -> [_ w343]
    frame False {
    }
    frame True {
      n168 = case shown="No Error" w343 {
        frame No Error {
          n169 = invoke on="Invoke Node" class="VI" method="FP.Close"() -> ()  [unwired: 3 in, 3 out]
        }
        frame Error {
          n170 = invoke on="Invoke Node" class="VI" method="FP.Open"("Activate"=TRUE ("Activate?")) -> ()  [unwired: 4 in, 5 out]
        }
      }
    }
  }
  n171 = local write "Module Admin"(w3) -> ()
